vi "Format to string.vi"(8 "error in (no error)":errorcluster, 11 "address":refnum<class "IPv4 Network Address.lvclass">) -> (0 "error out":errorcluster, 2 "address string":string, 3 "address out":refnum<class "IPv4 Network Address.lvclass">)   [LabVIEW 2020, in "NI_WFCN.lvlib" / "IPv4 Network Address.lvclass"]
doc: "Returns a human-readable string representation of this address."
uses:
  <vilib>/net/WFCN/Addressing/IPv4 Network Address/IPv4 Network Address.lvclass
  <vilib>/net/WFCN/Addressing/IPv4 Network Address/IPv4 Network Address.lvclass/IPv4 Network Address.ctl
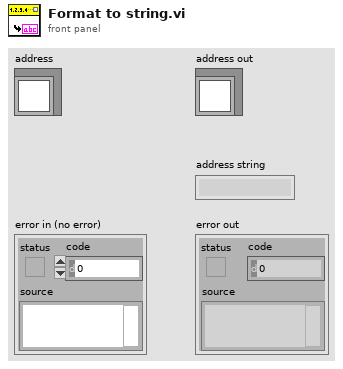
[diagram p1: front panel]
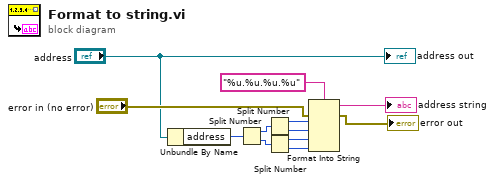
[diagram p0: block diagram]
diagram:
  n1 = Unbundle By Name("address") -> ("address"=w8:u32)
  n2 = Split Number(x=w8) -> (hi(x)=w7:u16, lo(x)=w6:u16)
  n3 = Split Number(x=w7) -> (hi(x)=w4:u8, lo(x)=w3:u8)
  n4 = Split Number(x=w6) -> (hi(x)=w2:u8, lo(x)=w1:u8)
  n5 = Format Into String(format string="%u.%u.%u.%u", error in="error in (no error)", w4, w3, w2, w1) -> (resulting string=→"address string":string, error out=→"error out":errorcluster)  [unwired: 1 in]
  "address out" <- "address"
